vi "change.volume.types.vi"(8 "error in (no error)":errorcluster, 9 "change criteria":T2, 11 "manager_daemon in":refnum<class "manager_daemon.lvclass">) -> (0 "error out":errorcluster, 2 "changed volume ids":i32[](array[numeric]), 3 "manager_daemon out":refnum<class "manager_daemon.lvclass">)   [LabVIEW 2024, in "manager_daemon.lvclass"]
uses:
  manager_daemon.lvclass
  CV_Shared_Library/volume.type--enum.ctl
  manager_daemon.lvclass/manager_daemon.ctl
  CV_Shared_Library/CV_Shared_Library.lvlib
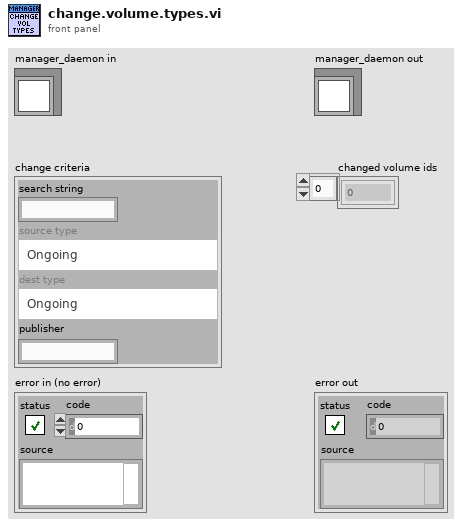
[diagram p1: front panel]
types:
  T1 = typedef "CV_Shared_Library.lvlib/volume.type--enum.ctl" = enum16{"Ongoing", "Limited Series", "Annual", "One Shot", "Reprint/Document", "Digital"}
  T2 = cluster{"search string":string, "source type":T1, "dest type":T1, "publisher":string}
  T3 = typedef "manager_daemon.lvclass/PublisherMap--map.ctl" = map{string, T4}
  T4 = typedef "manager_daemon.lvclass/PublisherData--cluster.ctl" = cluster{"id":i32, "volumes":set{i32}}
  T5 = typedef "manager_daemon.lvclass/VolumeData--cluster.ctl" = cluster{"name":string, "sortable_name":string, "aliases":string[], "description":string, "site_detail_url":string, "count_of_issues":i32, "start_year":i32, "publisher_id":i32, "issue_ids":i32[], "date_last_updated":timestamp, "volume":i32, "cv_id":string, "volume type":T1, "source_path":path}
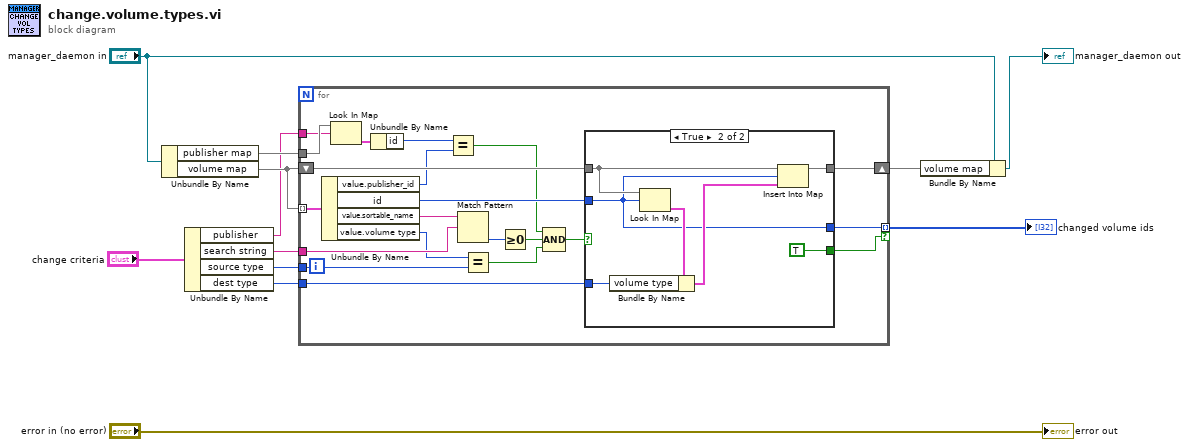
[diagram p0: block diagram]
diagram:
  n1 = Unbundle By Name("manager_daemon in") -> ("publisher map"=w2:T3, "volume map"=w9:map{i32, T5})
  n2 = Unbundle By Name("change criteria") -> ("publisher"=w1:string, "search string"=w11:string, "source type"=w10:T1, "dest type"=w5:T1)
  n3 = for {
    tunnel: w9 -> [w33] mode=indexing
    tunnel: w11 -> [w32]
    tunnel: w10 -> [w28]
    shift-right: [w23] -> w6
    shift-left: w9 -> [w24]
    tunnel: w5 -> [w21]
    tunnel: [w20] -> w3 mode=indexing if=w19
    tunnel: w2 -> [w18]
    tunnel: w1 -> [w17]
    n4 = Unbundle By Name(w33) -> ("value.publisher_id"=w14:i32, "id"=w22:i32, "value.sortable_name"=w31:string, "value.volume type"=w29:T1)
    n5 = Look In Map(map=w18, key=w17) -> (value=w16:T4)  [unwired: 1 in, 1 out]
    n6 = Unbundle By Name(w16) -> ("id"=w15:i32)
    n7 = Equal?(x=w15, y=w14) -> (x = y?=w13:bool)
    n8 = Match Pattern(string=w31, regular expression=w32) -> (offset past match=w30:i32)  [unwired: 1 in, 3 out]
    n9 = Equal?(x=w29, y=w28) -> (x = y?=w26:bool)
    n10 = Greater Or Equal To 0?(x=w30) -> (x >= 0?=w27:bool)
    n11 = Compound Arithmetic op=AND(w13, w27, w26) -> (w25:bool)
    n12 = case shown="True" w25 {
      tunnel: w24 -> [w34 w39]
      tunnel: [w34 w38] -> w23
      tunnel: w22 -> [_ w35]
      tunnel: w21 -> [_ w40]
      tunnel: [_ w35] -> w20
      tunnel: [_ TRUE] -> w19
      frame False {
      }
      frame True {
        n13 = Look In Map(map=w39, key=w35) -> (value=w41:T5)  [unwired: 1 in, 1 out]
        n14 = Bundle By Name(cluster=w41, "volume type"=w40) -> (w37:T5)
        n15 = Insert Into Map(map in=w39, key=w35, value=w37) -> (map out=w38:map{i32, T5})  [unwired: 2 out]
      }
    }
  }
  "changed volume ids" <- w3
  n16 = Bundle By Name(cluster="manager_daemon in", "volume map"=w6) -> (→"manager_daemon out":refnum<class "manager_daemon.lvclass">)
  "error out" <- "error in (no error)"
